vi "stringtoxmllist.vi"(1 "List of XML parameters to write":string[](array[string]), 2 "Channel On/Off Array":bool[](array[boolean]), 3 "List Name":string, 4 "Input String":string) -> (0 "concatenated string":string)   [LabVIEW 2012]
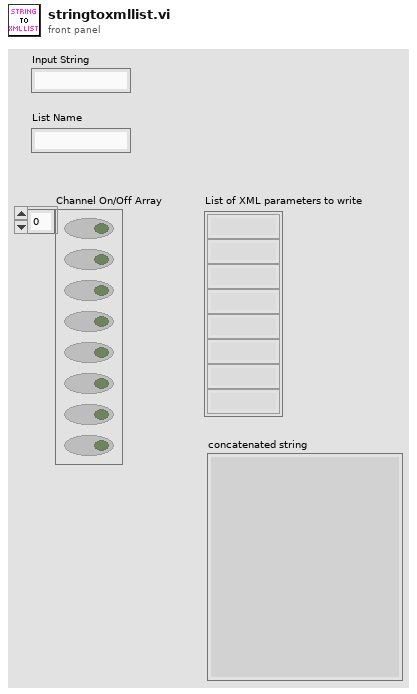
[diagram p1: front panel]
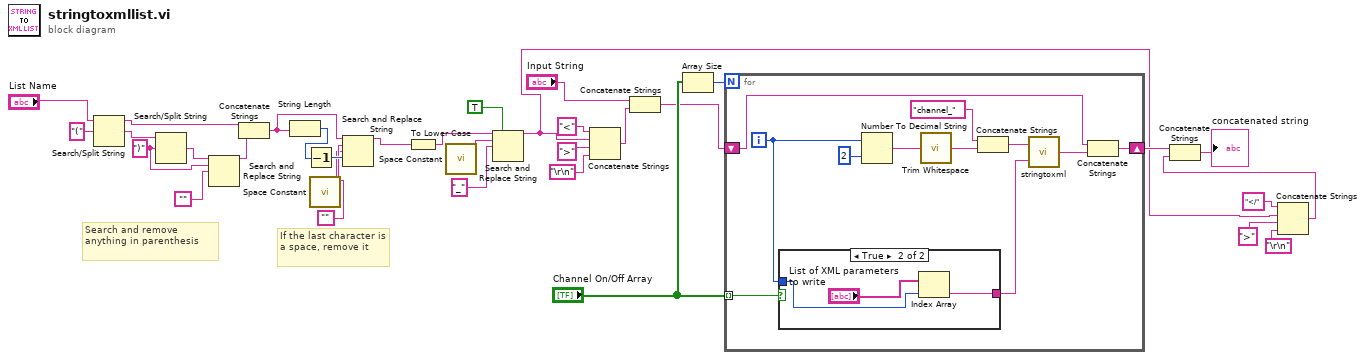
[diagram p0: block diagram]
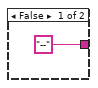
[diagram p2: hidden frame]
diagram:
  w10 = ")" ("search string/char (-)")
  # "If the last character is a space, remove it"
  # "Search and remove anything in parenthesis"
  n1 = Search/Split String(string="List Name", search string/char (-)="(") -> (substring before match=w13:string, match + rest of string=w14:string)  [unwired: 1 in, 1 out]
  n2 = Search/Split String(string=w14, search string/char (-)=w10) -> (match + rest of string=w12:string)  [unwired: 1 in, 2 out]
  n3 = Search and Replace String(input string=w12, search string=w10, replace string="") -> (result string=w9:string)  [unwired: 5 in, 3 out]
  n4 = Concatenate Strings(w13, w9) -> (w6:string)
  n5 = String Length(string=w6) -> (length=w8:i32)
  n6 = Decrement(x=w8) -> (x-1=w7:i32)
  n7 = call <vilib>:"Space Constant.vi"() -> ("String"=w5:string)
  n8 = Search and Replace String(input string=w6, search string=w5, replace string="", offset=w7) -> (result string=w2:string)  [unwired: 4 in, 3 out]
  n9 = To Lower Case(string=w2) -> (all lower case string=w19:string)
  n10 = call <vilib>:"Space Constant.vi"() -> ("String"=w17:string)
  n11 = Search and Replace String(replace all?=TRUE ("replace all? (F)"), input string=w19, search string=w17, replace string="_") -> (result string=w1:string)  [unwired: 4 in, 3 out]
  n12 = Concatenate Strings("<" ("string"), w1, ">" ("string"), "\r\n") -> (w21:string)
  n13 = Concatenate Strings("Input String", w21) -> (w20:string)
  n14 = Array Size(array="Channel On/Off Array") -> (size(s)=w23:i32)
  n15 = for {
    N: w23 -> [_]
    tunnel: "Channel On/Off Array" -> [w44] mode=indexing
    shift-right: [w37] -> w25
    shift-left: w20 -> [w39]
    i -> [w34]
    n16 = case shown="True" w44 {
      tunnel: w34 -> [_ w47]
      tunnel: ["--" ("String") w46] -> w40
      frame False {
      }
      frame True {
        n17 = Index Array(array="List of XML parameters to write", index=w47) -> (element=w46:string)
      }
    }
    n18 = Number To Decimal String(number=w34, width (-)=i16 2) -> (decimal integer string=w36:string)
    n19 = call <vilib>:"Trim Whitespace.vi"("string"=w36) -> ("trimmed string"=w35:string)  [unwired: 1 in]
    n20 = Concatenate Strings("channel_" ("initial string"), w35) -> (w41:string)
    n21 = call "stringtoxml.vi"("String to write"=w40, "XML Tag"=w41) -> ("xml string"=w38:string)
    n22 = Concatenate Strings(w39, w38) -> (w37:string)
  }
  n23 = Concatenate Strings("</" ("string"), w1, ">" ("string"), "\r\n") -> (w29:string)
  n24 = Concatenate Strings(w25, w29) -> (→"concatenated string":string)
